vi "PT Settings Dialog.vi"(8 "error in (no error)":errorcluster, 11 "PT Module Config in":T2) -> (0 "error out":errorcluster, 1 "Cancelled?":bool=TRUE, 2 "UI Refresh Needed?":bool, 3 "PT Module Config out":T2)   [LabVIEW 2018, in "PT Module.lvlib"]
doc: "Dialog for selecting user specified settings."
uses:
  PT Module.lvlib
  Controls/PT Module Config Cluster.ctl
  <vilib>/Utility/miscctls.llb/LVPoint32TypeDef.ctl
  Tag VIs/Numeric Alarm Settings Cluster.ctl
  Controls/PT Settings Dialog.ctl
  Tag VIs/Tag FGV Operation Enum.ctl
  Shared Variables/Simple Alarm Values Cluster.ctl
  Shared Variables/Dynamic Shared Variables.lvlib
panel:
  in  "Module Name":string
  in  "Settings Dialog":T1
  in  "Cancel Button":bool
  in  "OK Button":bool
  # "Non visible portion of dialog (needed for connector pane)."
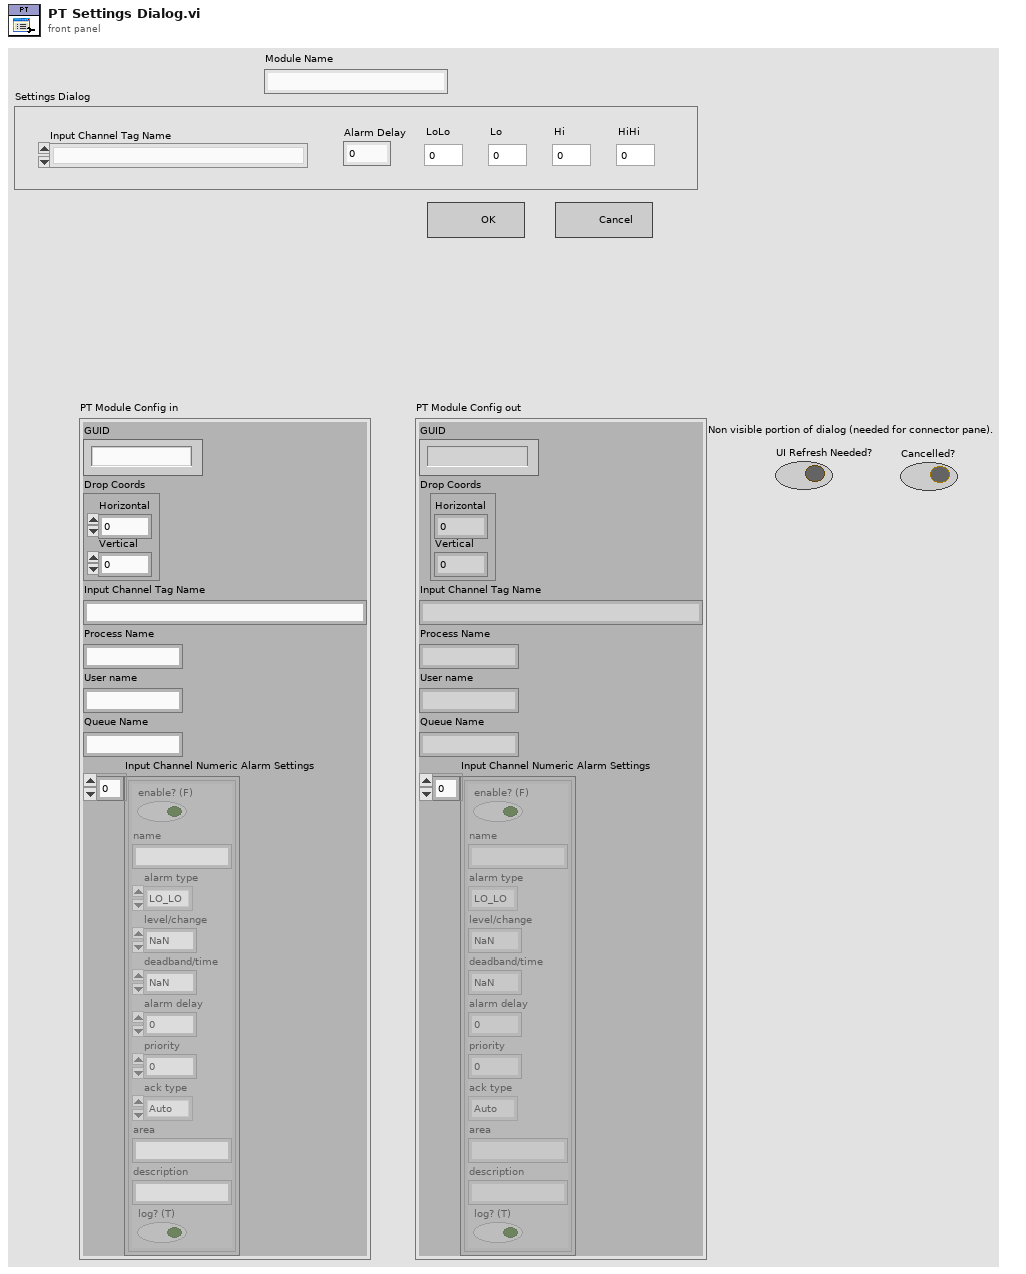
[diagram p1: front panel]
types:
  T1 = typedef "PT Module.lvlib/PT Settings Dialog.ctl" = cluster{"Input Channel Tag Name":u16, "LoLo":dbl, "Lo":dbl, "Hi":dbl, "HiHi":dbl, "Alarm Delay":dbl}
  T2 = typedef "PT Module.lvlib/PT Module Config Cluster.ctl" = cluster{"GUID":string, "Drop Coords":T3, "Input Channel Tag Name ":string, "Process Name":string, "User name":string, "Queue Name":string, "Input Channel Numeric Alarm Settings":T4[]}
  T3 = typedef "LVPoint32TypeDef.ctl" = cluster{"Horizontal":i32, "Vertical":i32}
  T4 = typedef "Numeric Alarm Settings Cluster.ctl" = cluster{"enable? (F)":bool, "name":string, "alarm type":enum16{"HI_HI", "HI", "LO", "LO_LO"}, "level/change":dbl, "deadband/time":dbl, "alarm delay":dbl, "priority":u32, "ack type":enum16{"Auto", "User", "None", "Each Occurrence"}, "area":string, "description":string, "log? (T)":bool}
  T5 = typedef "Tag FGV Operation Enum.ctl" = enum16{"Init", "Set Notification Queue", "Create Tag", "Commit", "Write Tag (Numeric)", "Write Tag (Boolean)", "Read All Tags", "Read One Tag", "Delete Tag Category", "Set Alarm Parameters (Numeric)", "Set Alarm Parameters (Boolean)", "Enable All Alarms", "Disable All Alarms", "Delete All Tags", "Read Alarms", "Ack Alarm", "Read Alarm Parameters (Numeric)", "Read Alarm Parameters (Boolean)"}
  T6 = typedef "Dynamic Shared Variables.lvlib/Simple Alarm Values Cluster.ctl" = cluster{"tag name":string, "HiHi":dbl, "Hi":dbl, "Lo":dbl, "LoLo":dbl, "alarm delay":dbl}
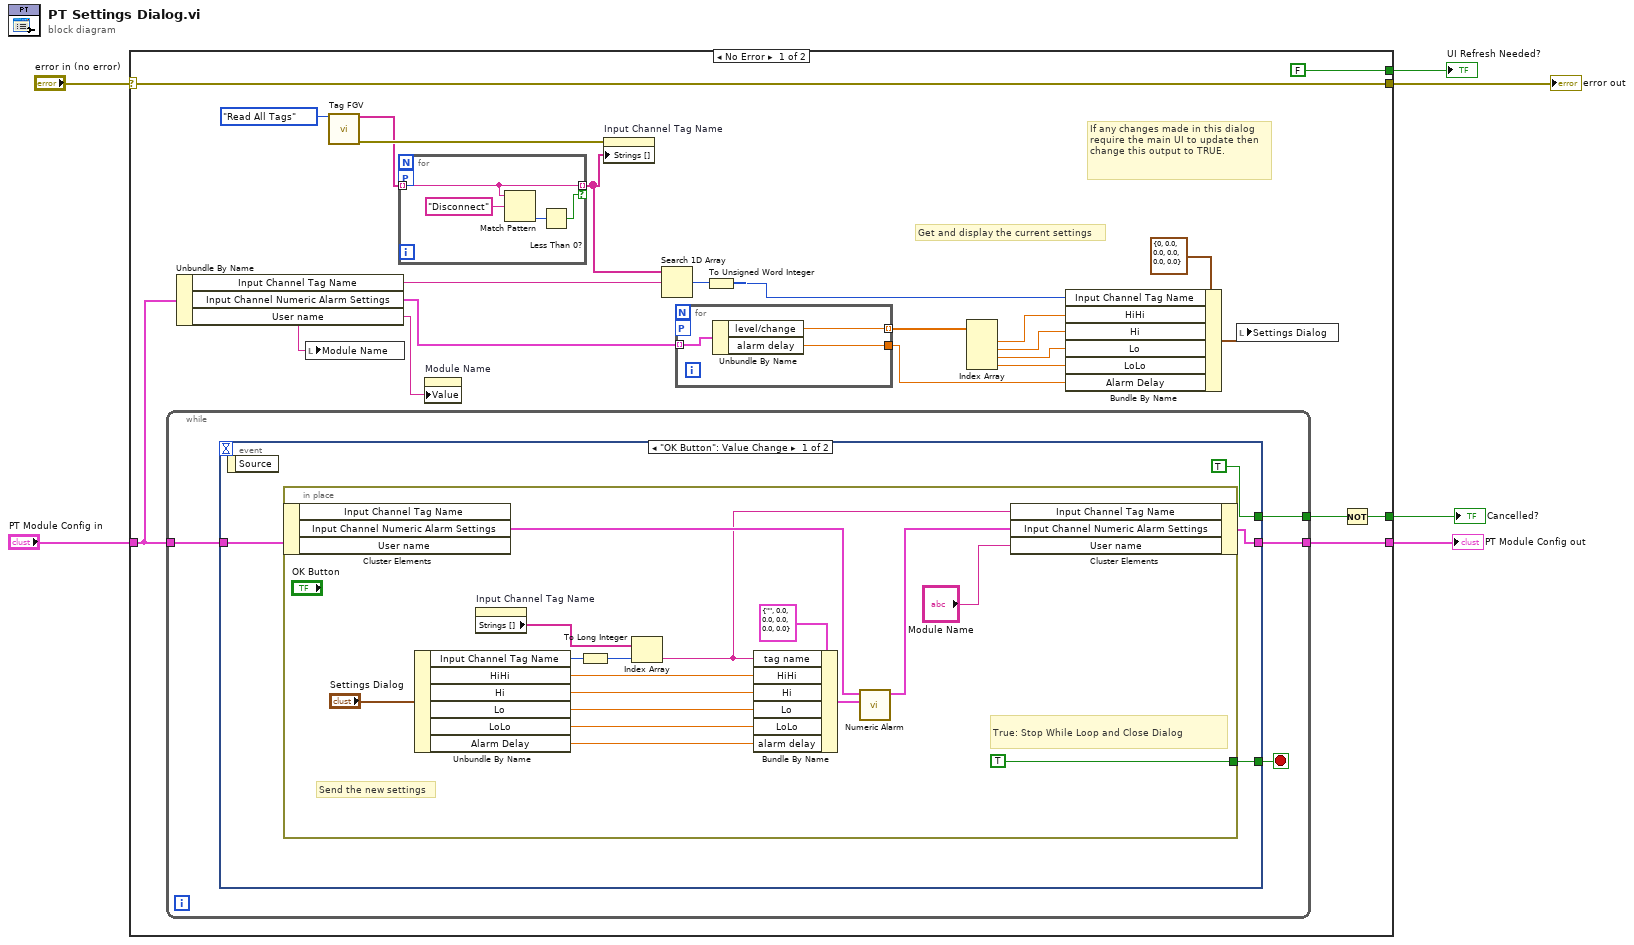
[diagram p0: block diagram]
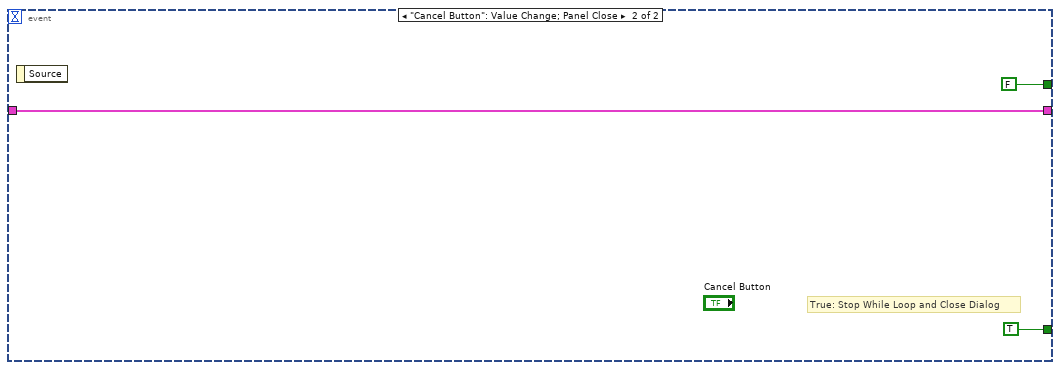
[diagram p2: hidden frame]
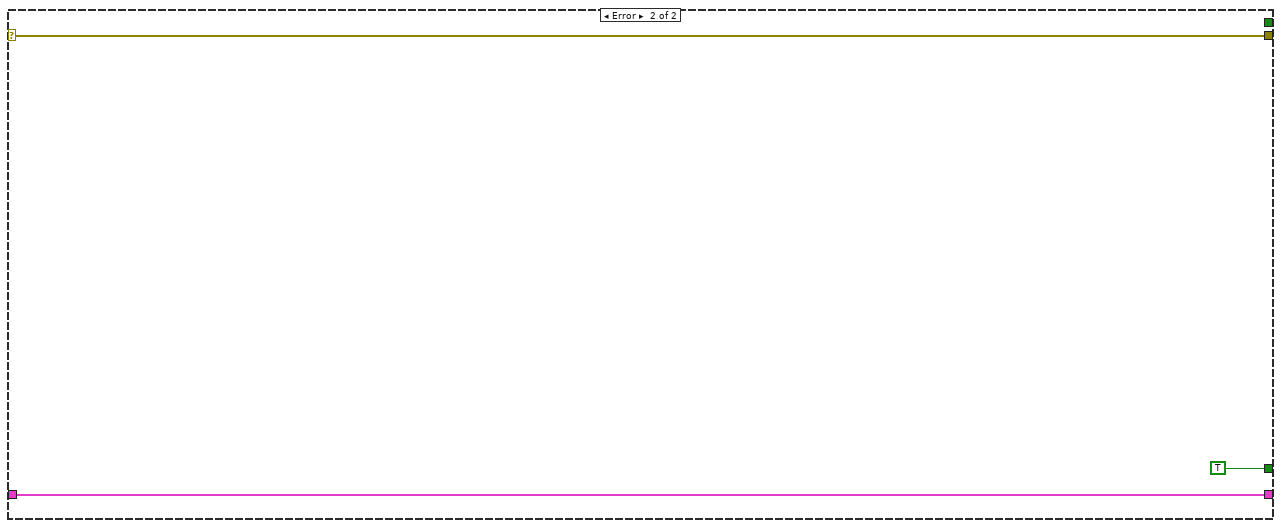
[diagram p3: hidden frame]
diagram:
  n1 = case shown="No Error" "error in (no error)" {
    selector: "error in (no error)" -> [w29 w66]
    tunnel: [w29 w66] -> w6
    tunnel: "PT Module Config in" -> [w26 w65]
    tunnel: [w27 w65] -> w1
    tunnel: [FALSE ("UI Refresh Needed?") _] -> w4
    tunnel: [w24 TRUE ("UI Refresh Needed?")] -> w3
    frame No Error {
      # "Get and display the current settings"
      # "If any changes made in this dialog require the main UI to update then change this output to TRUE."
      n2 = while {
        tunnel: [w40] -> w25
        tunnel: [w37] -> w27
        tunnel: w26 -> [w39]
        stop <- w38 stop-if-true
        n3 = event shown="[0] \"OK Button\": Value Change" {
          selector: _ -> [_ _]
          dyn-events: _ -> [_ _]
          timeout: _ -> [_ _]
          tunnel: w39 -> [w42 w63]
          tunnel: [TRUE ("UI Refresh Needed?") FALSE ("UI Refresh Needed?")] -> w40
          tunnel: [w43 TRUE] -> w38
          tunnel: [w41 w63] -> w37
          event "OK Button": Value Change {
            n4 = event-data() -> ()  [unwired: 1 in, 1 out]
            n5 = in-place {
              in-place-border: [TRUE] -> w43
              # "Send the new settings"
              # "True: Stop While Loop and Close Dialog"
              n6 = in-place-cluster #1(w42) -> ("Input Channel Numeric Alarm Settings"=w48:T4[])  [unwired: 2 out]
              n7 = Unbundle By Name("Settings Dialog") -> ("Input Channel Tag Name"=w58:u16, "HiHi"=w57:dbl, "Hi"=w56:dbl, "Lo"=w55:dbl, "LoLo"=w51:dbl, "Alarm Delay"=w49:dbl)
              n8 = property on="Input Channel Tag Name" class="Ring (strict)"() -> ("Strings []"=w59:string[])  [unwired: 2 in, 2 out]
              n9 = To Long Integer(number=w58) -> (32bit integer=w53:i32)
              n10 = Index Array(array=w59, index=w53) -> (element=w47:string)
              n11 = Bundle By Name(cluster=T6 {"tag name"="", "HiHi"=0.0, "Hi"=0.0, "Lo"=0.0, "LoLo"=0.0, "alarm delay"=0.0} ("Simple Alarm Values"), "tag name"=w47, "HiHi"=w57, "Hi"=w56, "Lo"=w55, "LoLo"=w51, "alarm delay"=w49) -> (w50:T6)
              n12 = call "Numeric Alarm.vi"("Simple Alarm Values"=w50, "Alarms in"=w48) -> ("Alarms out"=w46:T4[])  [unwired: 9 in]
              n13 = in-place-cluster #1("Input Channel Tag Name"=w47, "Input Channel Numeric Alarm Settings"=w46, "User name"="Module Name") -> (w41:T2)
            }
          }
          event "Cancel Button": Value Change; Panel Close {
            # "True: Stop While Loop and Close Dialog"
            n14 = event-data() -> ()  [unwired: 1 in, 1 out]
          }
        }
      }
      n15 = Unbundle By Name(w26) -> ("Input Channel Tag Name"=w21:string, "Input Channel Numeric Alarm Settings"=w13:T4[], "User name"=w10:string)
      n16 = local write "Module Name"(w10) -> ()
      n17 = call "Tag FGV.vi"("Operation"=Tag_FGV_Operation_Enum."Read All Tags") -> ("Tag Names"=w9:string[], "error out"=w23:errorcluster)  [unwired: 7 in, 6 out]
      n18 = for {
        tunnel: w9 -> [w31] mode=indexing
        tunnel: [w31] -> w8 mode=indexing if=w30
        workers-P: _ -> [_]
        n19 = Match Pattern(string=w31, regular expression="Disconnect" ("name")) -> (offset past match=w33:i32)  [unwired: 1 in, 3 out]
        n20 = Less Than 0?(x=w33) -> (x < 0?=w30:bool)
      }
      n21 = property on="Module Name" class="Str"("Value"=w10) -> ()  [unwired: 2 in, 2 out]
      n22 = property on="Input Channel Tag Name" class="Ring (strict)"(error in=w23, "Strings []"=w8) -> ()  [unwired: 1 in, 2 out]
      n23 = Search 1D Array(1D array=w8, element=w21) -> (index of element=w20:i32)  [unwired: 1 in]
      n24 = for {
        tunnel: w13 -> [w36] mode=indexing
        tunnel: [w35] -> w12 mode=indexing
        tunnel: [w34] -> w7
        workers-P: _ -> [_]
        n25 = Unbundle By Name(w36) -> ("level/change"=w35:dbl, "alarm delay"=w34:dbl)
      }
      n26 = To Unsigned Word Integer(number=w20) -> (unsigned 16bit integer=w11:u16)
      n27 = Index Array(array=w12) -> (element #1=w17:dbl, element #2=w16:dbl, element #3=w15:dbl, element #4=w14:dbl)  [unwired: 4 in]
      n28 = Bundle By Name(cluster=T1 {"Input Channel Tag Name"=0, "LoLo"=0.0, "Lo"=0.0, "Hi"=0.0, "HiHi"=0.0, "Alarm Delay"=0.0} ("Settings Dialog"), "Input Channel Tag Name"=w11, "HiHi"=w17, "Hi"=w16, "Lo"=w15, "LoLo"=w14, "Alarm Delay"=w7) -> (w18:T1)
      n29 = local write "Settings Dialog"(w18) -> ()
      n30 = Not(x=w25) -> (.not. x?=w24:bool)
    }
    frame Error {
    }
  }
  "UI Refresh Needed?" <- w4
  "error out" <- w6
  "PT Module Config out" <- w1
  "Cancelled?" <- w3
